vi "RemoteControl.TestLauncher.Server.vi"() -> ()   [LabVIEW 2016, in "RemoteControl.lvclass"]
uses:
  RemoteControl.lvclass
  <vilib>/JKI/JKI SMO/SMO/Typedefs/SMOState --Enum.ctl
  C:/Program Files (x86)/National Instruments/LabVIEW 2016/vi.lib/JKI/JKI SMO/SMO/SMO.lvclass
  RemoteControl.STM/RemoteControl.STM.lvclass
  C:/user/patrick/hg/levylab_util_remote/src/SMOs/RemoteControl/RemoteControl.lvclass
  <vilib>/JKI/JKI SMO/SMO/SMO.lvclass
panel:
  in  "T = STM":bool
  out "SMO State":T1
  out "error out":errorcluster
  in  "Stop":bool
  # "SM SMO Test Launcher: Server"
  # "UNUSED I THINK!!!!"
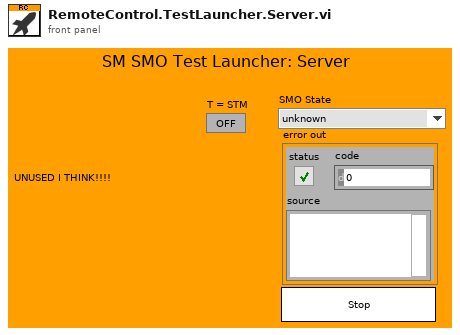
[diagram p1: front panel]
types:
  T1 = typedef "SMO.lvclass/SMOState --Enum.ctl" = enum16{"unknown", "Created", "Started", "Stopped"}
  T2 = typedef "SMO.lvclass/Public Events.ctl" = cluster{"Error":refnum<user-event>, "State":refnum<user-event>, "Reserve State":refnum<user-event>}
  T3 = typedef "RemoteControl.lvclass/PublicEvents--Cluster.ctl" = cluster{"SendMessageFromProcess":refnum<user-event>}
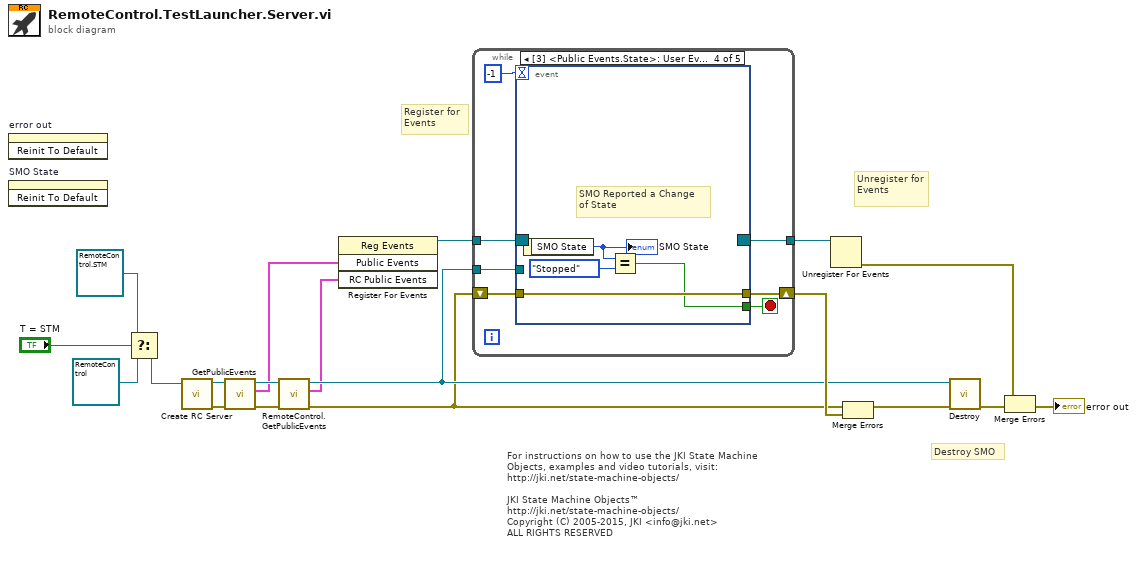
[diagram p0: block diagram]
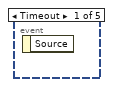
[diagram p2: hidden frame]
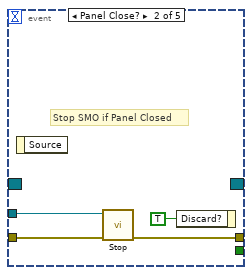
[diagram p3: hidden frame]
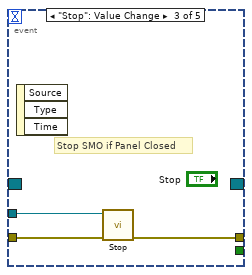
[diagram p4: hidden frame]
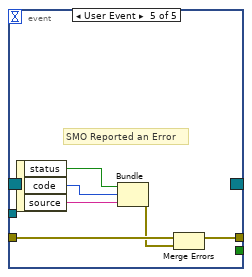
[diagram p5: hidden frame]
diagram:
  # "For instructions on how to use the JKI State Machine Objects, examples and video tutorials, visit:\nhttp://jki.net/state-machine-objects/\n\nJKI State Machine Objects™\nhttp://jki.net/state-machine-objects/\nCopyright (C) 2005-2015, JKI <info@jki.net>\nALL RIGHTS RESERVED"
  # "Destroy SMO"
  # "Unregister for Events"
  # "Register for Events"
  n1 = invoke on="error out" class="Clust (strict)" method="Reinit To Default"() -> ()  [unwired: 3 in, 3 out]
  n2 = invoke on="SMO State" class="Enum (strict)" method="Reinit To Default"() -> ()  [unwired: 3 in, 3 out]
  n3 = Select(t=refnum<class "RemoteControl.STM.lvclass"> refnum ("RemoteControl.STM.lvclass"), s="T = STM", f=refnum<class "RemoteControl.lvclass"> refnum ("SMO.Template.lvclass")) -> (s? t:f=w11:refnum<class "RemoteControl.lvclass">)
  n4 = call-dynamic "Create RC Server.vi"("RemoteControl in"=w11) -> ("error out"=w9:errorcluster, "RemoteControl out"=w8:refnum<class "RemoteControl.lvclass">)  [unwired: 9 in]
  n5 = call <vilib>:"GetPublicEvents.vi"("error in (no error)"=w9, "SMO"=w8) -> ("error out"=w7:errorcluster, "Public Events"=w2:T2, "SMO out"=w6:refnum<class "RemoteControl.lvclass">)  [unwired: 7 in]
  n6 = call "RemoteControl.GetPublicEvents.vi"("error in (no error)"=w7, "RemoteControl"=w6) -> ("error out"=w4:errorcluster, "RC Public Events"=w1:T3, "RemoteControl out"=w5:refnum<class "RemoteControl.lvclass">)  [unwired: 7 in]
  n7 = register-events(w2, w1) -> (reference out=w3:refnum<event-registration>)  [unwired: 2 in, 1 out]
  n8 = while {
    shift-right: [w25] -> w18
    shift-left: w4 -> [w24]
    tunnel: w3 -> [w23]
    tunnel: [w22] -> w19
    tunnel: w5 -> [w21]
    stop <- w26 stop-if-true
    n9 = event shown="[3] <Public Events.State>: User Event" {
      selector: w23 -> [_ _ _ _ _]
      dyn-events: [_ _ _ _ _] -> w22
      timeout: -1 -> [_ _ _ _ _]
      tunnel: [_ _ _ w34 _] -> w26
      tunnel: w21 -> [_ w30 w33 _ _]
      tunnel: [_ w29 w32 w37 w41] -> w25
      tunnel: w24 -> [_ w28 w31 w37 w39]
      event Timeout {
        n10 = event-data() -> ()  [unwired: 1 in, 1 out]
      }
      event Panel Close? {
        # "Stop SMO if Panel Closed"
        n11 = event-data() -> ()  [unwired: 1 in, 1 out]
        n12 = call <vilib>:"Stop.vi"("error in (no error)"=w28, "SMO"=w30) -> ("error out"=w29:errorcluster)  [unwired: 8 in, 1 out]
        n13 = event-data("Discard?"=TRUE ("OK")) -> ()  [unwired: 1 in, 1 out]
      }
      event "Stop": Value Change {
        # "Stop SMO if Panel Closed"
        n14 = event-data() -> ()  [unwired: 1 in, 3 out]
        n15 = call <vilib>:"Stop.vi"("error in (no error)"=w31, "SMO"=w33) -> ("error out"=w32:errorcluster)  [unwired: 8 in, 1 out]
      }
      event User Event {
        # "SMO Reported a Change\nof State"
        n16 = event-data() -> ("SMO State"=w36:T1)  [unwired: 1 in]
        "SMO State" <- w36
        n17 = Equal?(x=w36, y=SMOState_--Enum."Stopped") -> (x = y?=w34:bool)
      }
      event User Event {
        # "SMO Reported an Error"
        n18 = event-data() -> ("status"=w40:bool, "code"=w43:i32, "source"=w42:string)  [unwired: 1 in]
        n19 = Bundle("status"=w40, "code"=w43, "source"=w42) -> (w38:errorcluster)  [unwired: 1 in]
        n20 = Merge Errors(w39, w38) -> (w41:errorcluster)
      }
    }
  }
  n21 = Unregister For Events(event registration refnum=w19) -> (error out=w17:errorcluster)  [unwired: 1 in]
  n22 = Merge Errors(w4, w18) -> (w14:errorcluster)
  n23 = call <vilib>:"Destroy.vi"("error in (no error)"=w14, "SMO"=w5) -> ("error out"=w15:errorcluster)  [unwired: 9 in]
  n24 = Merge Errors(w17, w15) -> (→"error out":errorcluster)
